vi "Conversor-bin-hex.vi"(11 "Numeric":i16) -> (0 "hex integer string":string, 3 "hex integer string 2":string)   [LabVIEW 2019]
panel:
  out "subarray 2":bool[](array[boolean])
  out "subarray":bool[](array[boolean])
  out "number 2":u32
  out "number":u32
  out "Boolean array":bool[](array[boolean])
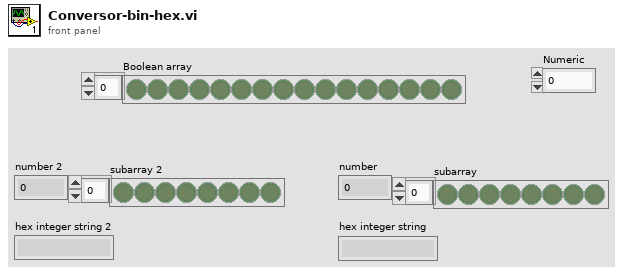
[diagram p1: front panel]
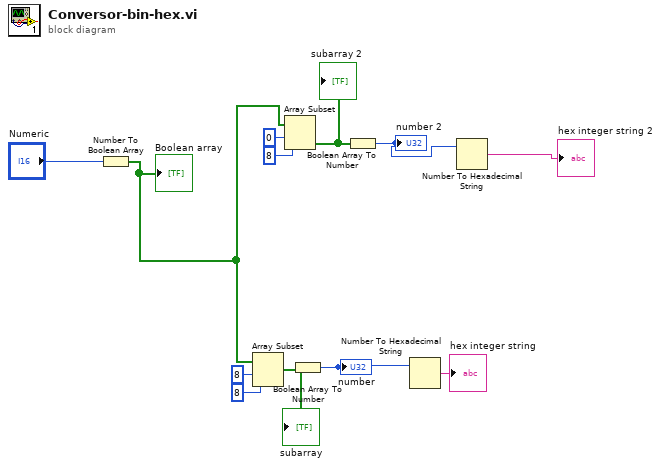
[diagram p0: block diagram]
diagram:
  n1 = Number To Boolean Array(number="Numeric") -> (Boolean array=w7:bool[])
  "Boolean array" <- w7
  n2 = Array Subset(array=w7, index=8, length=8) -> (w6:bool[])
  "subarray" <- w6
  n3 = Array Subset(array=w7, index=0, length=8) -> (w5:bool[])
  "subarray 2" <- w5
  n4 = Boolean Array To Number(Boolean array=w6) -> (number=w3:u32)
  "number" <- w3
  n5 = Boolean Array To Number(Boolean array=w5) -> (number=w4:u32)
  "number 2" <- w4
  n6 = Number To Hexadecimal String(2:w3) -> (0:→"hex integer string":string)  [unwired: 1 in]
  n7 = Number To Hexadecimal String(2:w4) -> (0:→"hex integer string 2":string)  [unwired: 1 in]
